vi "Find Controls and Indicators refs.vi"(11 "Ctrls[]":refnum<vi>[](array[refnum])) -> (2 "Controls Refs":refnum<vi>[](array[refnum]), 3 "Indicators Refs":refnum<vi>[](array[refnum]))   [LabVIEW 2020, in "DQMH_API.lvlib"]
uses:
  DQMH_API.lvlib
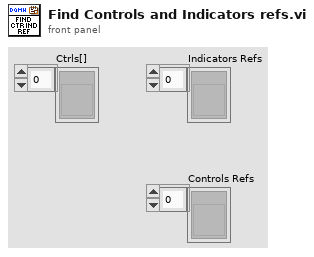
[diagram p1: front panel]
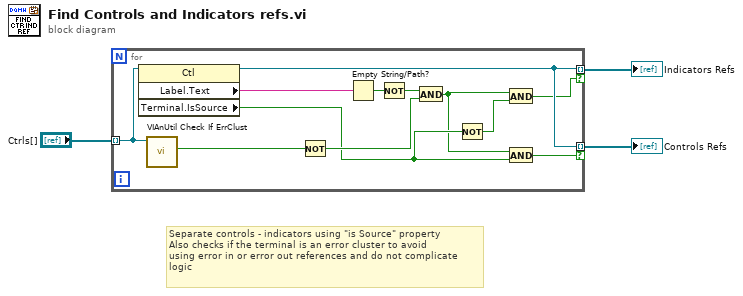
[diagram p0: block diagram]
diagram:
  # "Separate controls - indicators using \"is Source\" property\nAlso checks if the terminal is an error cluster to avoid\nusing error in or error out references and do not complicate\nlogic"
  n1 = for {
    tunnel: "Ctrls[]" -> [w10] mode=indexing
    tunnel: [w9] -> w2 mode=indexing if=w5
    tunnel: [w9] -> w3 mode=indexing if=w4
    n2 = property class="Ctl"(reference=w10) -> (reference out=w9:refnum<vi>, "Label.Text"=w13:string, "Terminal.IsSource"=w8:bool)  [unwired: 1 in, 1 out]
    n3 = call <vilib>:"VIAnUtil Check If ErrClust.vi"("Control in"=w10) -> ("Is error cluster?"=w12:bool)  [unwired: 8 in, 2 out]
    n4 = Not(x=w12) -> (.not. x?=w11:bool)
    n5 = Empty String/Path?(string/path=w13) -> (empty?=w15:bool)
    n6 = Not(x=w15) -> (.not. x?=w14:bool)
    n7 = And(x=w14, y=w11) -> (x .and. y?=w7:bool)
    n8 = Not(x=w8) -> (.not. x?=w6:bool)
    n9 = And(x=w7, y=w6) -> (x .and. y?=w5:bool)
    n10 = And(x=w7, y=w8) -> (x .and. y?=w4:bool)
  }
  "Controls Refs" <- w3
  "Indicators Refs" <- w2
